vi "Write Data.vi"(8 "error in":errorcluster, 10 "CRDS Cell":refnum<class "CRDS Cell Data.lvclass">, 11 "CRDS Cell in":refnum<class "CRDS Cell.lvclass">) -> (0 "error out":errorcluster, 3 "CRDS Cell out":refnum<class "CRDS Cell.lvclass">)   [LabVIEW 2016, in "CRDS Lib.lvlib" / "CRDS Cell.lvclass"]
uses:
  CRDS Cell.lvclass
  Data/Cell/CRDS Cell Data.lvclass
  CRDS Cell.lvclass/CRDS Cell.ctl
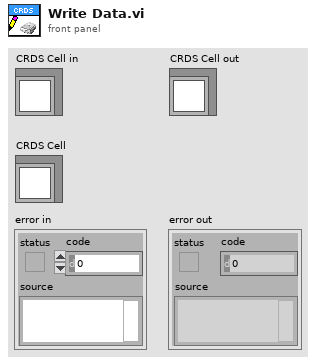
[diagram p1: front panel]
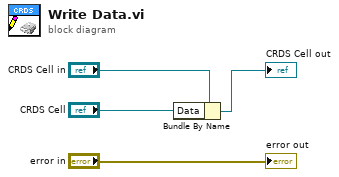
[diagram p0: block diagram]
diagram:
  n1 = Bundle By Name(cluster="CRDS Cell in", "Data"="CRDS Cell") -> (→"CRDS Cell out":refnum<class "CRDS Cell.lvclass">)
  "error out" <- "error in"
